vi "Multi Frequency Player.vi"() -> ()   [LabVIEW 2016]
uses:
  <vilib>/sound2/lvsound2.llb/Sound Data Format.ctl
  <vilib>/Platform/TimedLoop/XDataNode/timing_clust.ctl
  <vilib>/Platform/TimedLoop/XDataNode/nitl_modes.ctl
  <vilib>/Platform/TimedLoop/XDataNode/wakeup.ctl
  <vilib>/express/express analysis/Spectral/Block/exnSpectralBlock spectral measurements RMS poly.vi
  <vilib>/express/express analysis/Spectral/Block/exnSpectralBlock spectral measurements RMS WFM.vi
  <vilib>/sound2/lvsound2.llb/Sound Output Write (DBL Single).vi
  <vilib>/Platform/TimedLoop/XDataNode/XDataNode.xnode
  <vilib>/express/express analysis/Spectral/XNode/ExpressSpectralMeasurementsBlockNode.xnode
  <vilib>/measure/NI_MABase.lvlib
  <vilib>/Platform/TimedLoop/XDataNode/XDNodeRunTimeDep.lvlib
panel:
  in  "Volume":dbl(knob)=26.092426552014715 scale=0.0..100.0
  in  "Signals":T1(array[cluster])=[{"Amplitude (0-1)"={0.0, 1.0}, "Frequency (Hz)"=261.63}, {"Amplitude (0-1)"={0.0, 0.0}, "Frequency (Hz)"=277.18}, {"Amplitude (0-1)"={0.0, 0.0}, "Frequency (Hz)"=293.66}, {"Amplitude (0-1)"={0.0, 0.0}, "Frequency (Hz)"=311.13}, {"Amplitude (0-1)"={0.0, 1.0}, "Frequency (Hz)"=329.63}, {"Amplitude (0-1)"={0.014084507042253521, 0.0}, "Frequency (Hz)"=349.23}, {"Amplitude (0-1)"={0.0, 0.0}, "Frequency (Hz)"=369.99}, {"Amplitude (0-1)"={0.0, 1.0}, "Frequency (Hz)"=392.0}, {"Amplitude (0-1)"={0.0, 0.0}, "Frequency (Hz)"=415.3}, {"Amplitude (0-1)"={0.0, 0.0}, "Frequency (Hz)"=440.0}, {"Amplitude (0-1)"={0.0, 0.0}, "Frequency (Hz)"=466.16}, {"Amplitude (0-1)"={0.0, 0.0}, "Frequency (Hz)"=493.88}, {"Amplitude (0-1)"={0.0, 0.0}, "Frequency (Hz)"=523.25}] {"Amplitude (0-1)" scale=0.0..1.0}
  in  "Noise":cluster{"Type":u16, "Noise Amplitude":dbl}={"Type"=0, "Noise Amplitude"=0.5} {"Noise Amplitude" min=0.0 max=1.0 scale=0.0..1.0; "Type" items=["No Noise", "White Noise (uniform)", "Pink Noise (1/f)"]}
  in  "Filter":T2={"Type"=0, "Low Frequency\nCutoff (Hz)"=200.0, "High Frequency\nCutoff (Hz)"=400.0} {"Type" items=["No Filter", "Smoothing", "Highpass", "Lowpass", "Bandpass"]}
  in  "Note Duration (seconds)":dbl=4.0
  in  "device ID":u32
  out "Frequency Domain Signal":cluster{"f0":dbl, "df":dbl, "magnitude":dbl[]}(graph)={"f0"=0.0, "df"=0.25, "magnitude"=array[88200 elements]}
  out "Time Domain Signal":waveform(dbl)(graph)={"t0"=timestamp(0 s since 1904-01-01), "dt"=2.2675736961451248e-05, "Y"=array[176400 elements]} caption="Sine"
  # "Amplitude"
  # "Frequency"
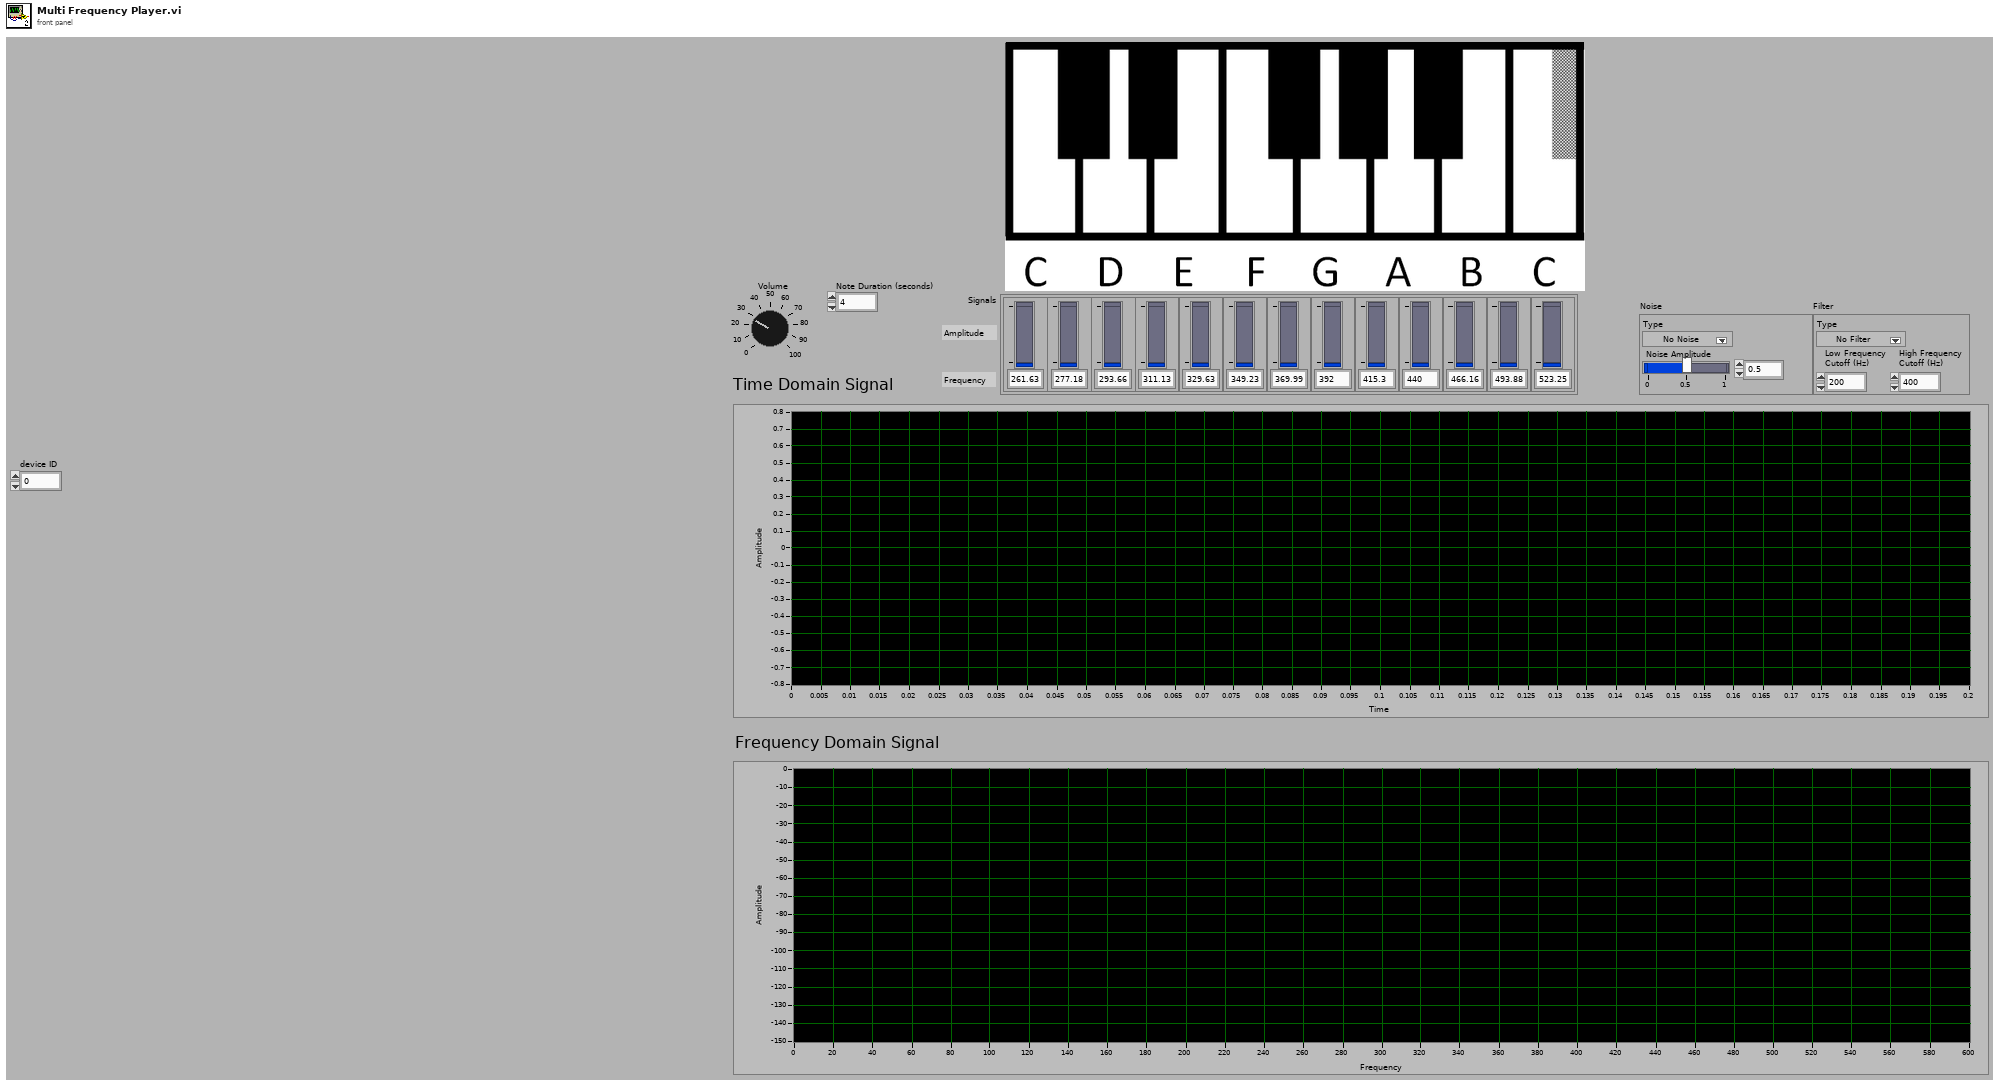
[diagram p1: front panel]
types:
  T1 = cluster{"Amplitude (0-1)":cluster{dbl, dbl}, "Frequency (Hz)":dbl}[]
  T2 = cluster{"Type":u16, "Low Frequency\nCutoff (Hz)":dbl, "High Frequency\nCutoff (Hz)":dbl}
  T3 = typedef "Sound Data Format.ctl" = cluster{"sample rate (S/s)":dbl, "number of channels":i32, "bits per sample":i32}
  T4 = typedef "Sound Output Task ID.ctl" = u32
  T5 = typedef "XDNodeRunTimeDep.lvlib/timing_clust.ctl" = cluster{"Expected End [f-1]":u64, "Actual End [f-1]":u64, "Finished Late? [f-1]":bool, "Expected End [i-1]":u64, "Actual End [i-1]":u64, "Finished Late? [i-1]":bool, "Expected Start [i]":u64, "Actual Start [i]":u64, "Expected Start [f]":u64, "Actual Start [f]":u64, "Source Name":string, "Structure Name":string, "Period":i64, "Deadline":i64, "Offset":i64, "Start":i64, "Priority":i32, "Timeout":i32, "Mode":T6, "Wakeup Reason":T7, "Error":errorcluster, "Source Type":string, "Secondary Source Type":string, "Global End Time":u64, "Global Start Time":u64, "Frame Duration":u64, "Iteration Duration":u64, "Assigned CPU":i32, "I/O Scan Engine Mode":u32}
  T6 = typedef "XDNodeRunTimeDep.lvlib/nitl_modes.ctl" = enum32{"No Change", "Process missed periods, maintain original phase", "Discard missed periods, maintain original phase", "Process missed periods, ignore original phase", "Discard missed periods, ignore original phase"}
  T7 = typedef "XDNodeRunTimeDep.lvlib/wakeup.ctl" = enum32{"Normal", "Aborted", "Asynchronous wakeup", "Timing source error", "Timed loop error", "Timeout"}
  T8 = cluster{"lower cutoff freq":dbl, "higher cutoff freq":dbl, "order":i32}
  T9 = cluster{"averaging mode":u16, "weighting mode":u16, "number of averages":u32}
  T10 = cluster{"dB On (F)":bool, "unwrap phase (F)":bool, "convert to degree (F)":bool}
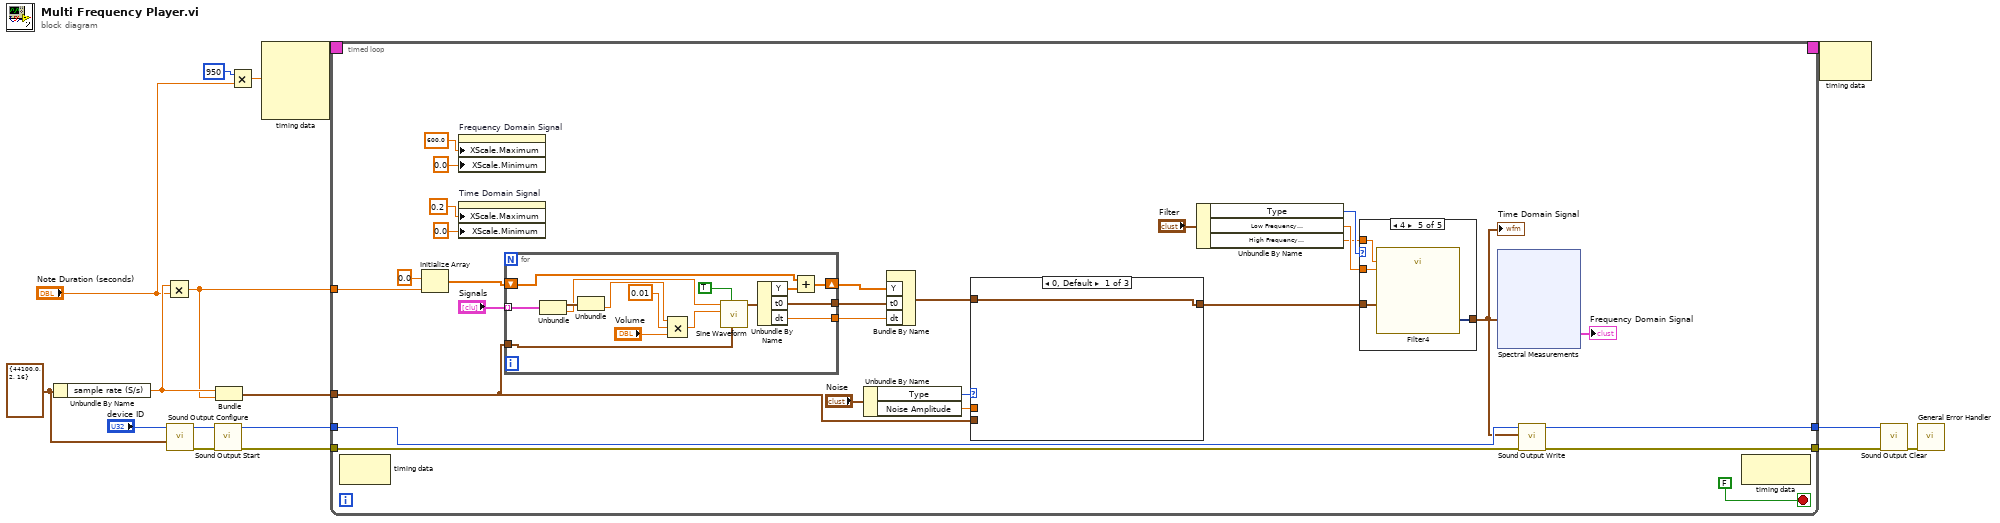
[diagram p0: block diagram]
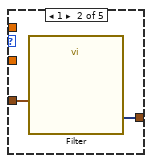
[diagram p3: hidden frame]
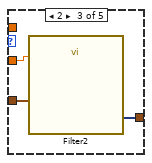
[diagram p4: hidden frame]
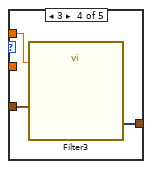
[diagram p5: hidden frame]
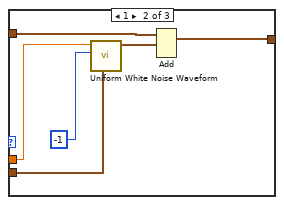
[diagram p6: hidden frame]
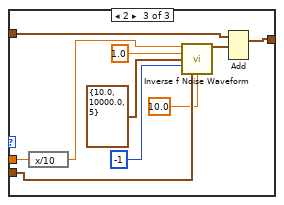
[diagram p7: hidden frame]
diagram:
  w14 = T3 {"sample rate (S/s)"=44100.0, "number of channels"=2, "bits per sample"=16} ("sound format")
  n1 = Unbundle By Name(w14) -> ("sample rate (S/s)"=w5:dbl)
  n2 = Multiply(x=w5, y="Note Duration (seconds)") -> (x*y=w4:dbl)
  n3 = call <vilib>:"Sound Output Configure.vi"("sound format"=w14, "device ID"="device ID") -> ("error out"=w15:errorcluster, "task ID"=w16:T4)  [unwired: 8 in]
  n4 = call <vilib>:"Sound Output Start.vi"("error in (no error)"=w15, "task ID"=w16) -> ("error out"=w11:errorcluster, "task ID out"=w12:T4)  [unwired: 8 in]
  n5 = Bundle("sample rate (S/s)"=w5, w4) -> (w6:cluster{"sample rate (S/s)":dbl, dbl})  [unwired: 1 in]
  n6 = Multiply(x=i64 950 ("Period"), y="Note Duration (seconds)") -> (x*y=w2:dbl)
  n7 = node-c288(w2) -> (w8:T5)  [unwired: 3 in]
  n8 = timed-loop {
    tunnel: w12 -> [w38]
    tunnel: w11 -> [w37]
    tunnel: [w36] -> w10
    tunnel: [w35] -> w9
    timing: w8 -> [_]
    timing-out: [_] -> w7
    tunnel: w6 -> [w33]
    tunnel: w4 -> [w27]
    stop <- FALSE stop-if-true
    n9 = node-c288() -> ()  [unwired: 1 in, 1 out]
    n10 = Initialize Array(0.0 ("element"), w27) -> (w32:dbl[])
    n11 = property on="Frequency Domain Signal" class="WFGraph (strict)"("XScale.Maximum"=600.0 ("X Scale.Range:Maximum"), "XScale.Minimum"=0.0 ("X Scale.Range:Minimum")) -> ()  [unwired: 2 in, 2 out]
    n12 = property on="Time Domain Signal" class="WFGraph (strict)"("XScale.Maximum"=0.2 ("X Scale.Range:Maximum"), "XScale.Minimum"=0.0 ("X Scale.Range:Minimum")) -> ()  [unwired: 2 in, 2 out]
    n13 = for {
      tunnel: w33 -> [w60]
      shift-right: [w55] -> w31
      shift-left: w32 -> [w57]
      tunnel: [w54] -> w29
      tunnel: [w53] -> w30
      tunnel: "Signals" -> [w52] mode=indexing
      n14 = Unbundle(w52) -> ("Amplitude (0-1)"=w51:cluster{dbl, dbl}, "Frequency (Hz)"=w50:dbl)
      n15 = Unbundle(w51) -> (w47:dbl)  [unwired: 1 out]
      n16 = Compound Arithmetic op=MULTIPLY(w47, 0.01 ("value"), "Volume") -> (w46:dbl)
      n17 = call <vilib>:"Sine Waveform.vi"("sampling info"=w60, "reset signal"=TRUE, "amplitude"=w46, "frequency"=w50) -> ("signal out"=w58:waveform(dbl))  [unwired: 6 in, 1 out]
      n18 = Unbundle By Name(w58) -> ("Y"=w56:dbl[], "t0"=w54:timestamp, "dt"=w53:dbl)
      n19 = Add(x=w57, y=w56) -> (x+y=w55:dbl[])
    }
    n20 = Unbundle By Name("Noise") -> ("Type"=w20:u16, "Noise Amplitude"=w19:dbl)
    n21 = Bundle By Name("Y"=w31, "t0"=w29, "dt"=w30) -> (w28:waveform(dbl))  [unwired: 1 in]
    n22 = case shown="0, Default" w20 {
      tunnel: [w76 w81 w90] -> w42
      tunnel: w28 -> [w76 w82 w92]
      tunnel: w33 -> [_ w78 w87]
      tunnel: w19 -> [_ w77 w84]
      frame 0, Default {
      }
      frame 1 {
        n23 = call <vilib>:"Uniform White Noise Waveform.vi"("sampling info"=w78, "seed"=-1, "amplitude"=w77) -> ("signal out"=w80:waveform(dbl))  [unwired: 7 in, 1 out]
        n24 = Add(1:w80, 2:w82) -> (0:w81:waveform(dbl))  [unwired: 1 in, 1 out]
      }
      frame 2 {
        n25 = expression code="x/10"(w84) -> (w83:dbl)
        n26 = call <vilib>:"Inverse f Noise Waveform.vi"("noise density"=w83, "exponent"=1.0, "filter specifications"=T8 {"lower cutoff freq"=10.0, "higher cutoff freq"=10000.0, "order"=5}, "seed"=-1, "sampling info"=w87, "reference freq (Hz)"=10.0) -> ("signal out"=w91:waveform(dbl))  [unwired: 5 in, 4 out]
        n27 = Add(1:w91, 2:w92) -> (0:w90:waveform(dbl))  [unwired: 1 in, 1 out]
      }
    }
    n28 = Unbundle By Name("Filter") -> ("Type"=w24:u16, "Low Frequency\nCutoff (Hz)"=w23:dbl, "High Frequency\nCutoff (Hz)"=w22:dbl)
    n29 = case shown="4" w24 {
      tunnel: [w63 w64 w67 w70 w72] -> w34
      tunnel: w42 -> [w63 w65 w68 w71 w73]
      tunnel: w23 -> [_ _ w66 _ w74]
      tunnel: w22 -> [_ _ _ w69 w75]
      frame 0, Default {
      }
      frame 1 {
        n30 = call "Filter"("Signal"=w65) -> ("Filtered Signal"=w64:dynamicdata)  [unwired: 9 in, 1 out]
      }
      frame 2 {
        n31 = call "Filter2"("Lower Cut-Off"=w66, "Signal"=w68) -> ("Filtered Signal"=w67:dynamicdata)  [unwired: 8 in, 1 out]
      }
      frame 3 {
        n32 = call "Filter3"("Lower Cut-Off"=w69, "Signal"=w71) -> ("Filtered Signal"=w70:dynamicdata)  [unwired: 8 in, 1 out]
      }
      frame 4 {
        n33 = call "Filter4"("Lower Cut-Off"=w74, "Upper Cut-Off"=w75, "Signal"=w73) -> ("Filtered Signal"=w72:dynamicdata)  [unwired: 7 in, 1 out]
      }
    }
    "Time Domain Signal" <- w34
    n34 = xnode "Spectral Measurements"("Signals"=w34) -> ("FFT - (RMS)"=→"Frequency Domain Signal":cluster{"f0":dbl, "df":dbl, "magnitude":dbl[]})  [unwired: 1 in, 2 out]
    n35 = call-poly <vilib>:"Sound Output Write.vi"("error in (no error)"=w37, "data"=w34, "task ID"=w38) -> ("error out"=w35:errorcluster, "task ID out"=w36:T4)  [unwired: 7 in]
    n36 = node-c288() -> ()  [unwired: 1 in, 1 out]
  }
  n37 = node-c288(w7) -> ()  [unwired: 1 out]
  n38 = call <vilib>:"Sound Output Clear.vi"("error in (no error)"=w9, "task ID"=w10) -> ("error out"=w13:errorcluster)  [unwired: 9 in]
  n39 = call <vilib>:"General Error Handler.vi"("error in (no error)"=w13) -> ()  [unwired: 2 in, 13 out]
